vi "Get check if at destination.vi"(8 "error in (no error)":errorcluster, 11 "StageSPIM in":refnum<class "StageSPIM.lvclass">) -> (0 "error out":errorcluster, 2 "check if at destination":bool, 3 "StageSPIM out":refnum<class "StageSPIM.lvclass">)   [LabVIEW 2012, in "StageSPIM.lvclass"]
uses:
  StageSPIM.lvclass
  Global check.vi
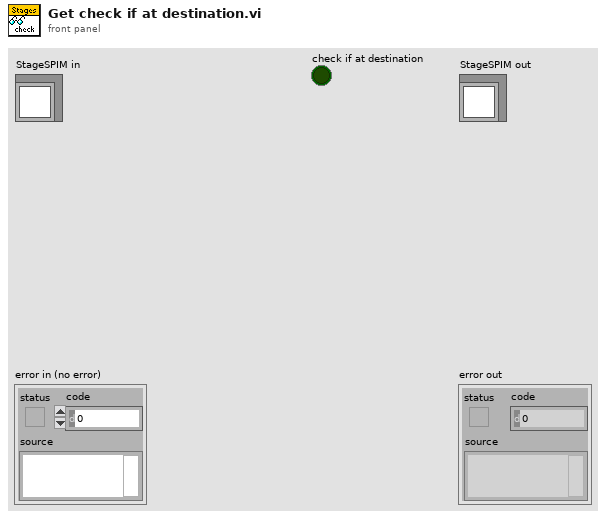
[diagram p1: front panel]
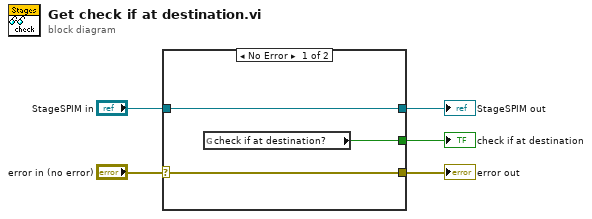
[diagram p0: block diagram]
diagram:
  n1 = case shown="No Error" "error in (no error)" {
    selector: "error in (no error)" -> [w8 w10]
    tunnel: [w8 w10] -> w4
    tunnel: [w7 w9] -> w2
    tunnel: "StageSPIM in" -> [w7 w9]
    tunnel: [w6 _] -> w1
    frame No Error {
      n2 = global read "Global check.vi" "check if at destination?"() -> (w6:bool)
    }
    frame Error {
    }
  }
  "error out" <- w4
  "StageSPIM out" <- w2
  "check if at destination" <- w1
